vi "FuzzyEx Car Backward Parking.vi"() -> ()   [LabVIEW 2018]
doc: "本范例演示使用模糊逻辑在指定位置停车。"
uses:
  <vilib>/addons/Fuzzy Logic/TypeDefs/FL System.ctl
  <vilib>/addons/Fuzzy Logic/TypeDefs/FL Variable.ctl
  <vilib>/addons/Fuzzy Logic/TypeDefs/FL Membership Function.ctl
  <vilib>/addons/Fuzzy Logic/TypeDefs/FL Membership Function Shape.ctl
  <vilib>/addons/Fuzzy Logic/TypeDefs/FL Rule.ctl
  <vilib>/addons/Fuzzy Logic/TypeDefs/FL Antecedent.ctl
  <vilib>/addons/Fuzzy Logic/TypeDefs/FL Modifier.ctl
  <vilib>/addons/Fuzzy Logic/TypeDefs/FL Antecedent Connective.ctl
  <vilib>/addons/Fuzzy Logic/TypeDefs/FL Consequent.ctl
  <vilib>/addons/Fuzzy Logic/TypeDefs/FL Consequent Implication.ctl
  <vilib>/addons/Fuzzy Logic/TypeDefs/FL Defuzzification.ctl
  <vilib>/addons/Fuzzy Logic/TypeDefs/FL Interpolating polynomials.ctl
  <vilib>/addons/Fuzzy Logic/FL Fuzzy Controller (MISO).vi
  <vilib>/addons/Fuzzy Logic/NI_Fuzzy_Logic_API.lvlib
panel:
  out "反向模糊系统":T1={"input variables"=[{"name"="汽车-位置", "range"=[0.0, 10.0, 0.0, 10.0], "MFs"=[{"name"="左", "shape"=1, "points"=[0.0, 0.0, 1.0, 4.0], "color"=16711680, "user-defined shape index"=0}, {"name"="左-中", "shape"=0, "points"=[3.0, 4.0, 5.0], "color"=3342438, "user-defined shape index"=0}, {"name"="中", "shape"=0, "points"=[4.5, 5.0, 5.5], "color"=255, "user-defined shape index"=0}, {"name"="右-中", "shape"=0, "points"=[5.0, 6.0, 7.0], "color"=16724991, "user-defined shape index"=0}, {"name"="右", "shape"=1, "points"=[6.0, 9.0, 10.0, 10.0], "color"=26214, "user-defined shape index"=0}]}, {"name"="汽车-方向", "range"=[-90.0, 270.0, -90.0, 270.0], "MFs"=[{"name"="左-下", "shape"=1, "points"=[-90.0, -90.0, -45.0, 20.000000000000014], "color"=16711680, "user-defined shape index"=0}, {"name"="左", "shape"=0, "points"=[-20.000000000000014, 20.000000000000014, 70.0], "color"=3342438, "user-defined shape index"=0}, {"name"="左-上", "shape"=0, "points"=[45.0, 70.0, 90.0], "color"=16724991, "user-defined shape index"=0}, {"name"="上", "shape"=0, "points"=[75.0, 90.0, 104.99999999999999], "color"=255, "user-defined shape index"=0}, {"name"="右-上", "shape"=0, "points"=[90.0, 110.0, 135.0], "color"=10040064, "user-defined shape index"=0}, {"name"="右", "shape"=0, "points"=[110.0, 160.0, 200.0], "color"=13056, "user-defined shape index"=0}, {"name"="右-下", "shape"=1, "points"=[160.0, 225.0, 270.0, 270.0], "color"=26214, "user-defined shape index"=0}]}], "output variables"=[{"name"="转向-角", "range"=[-30.0, 30.0, -30.0, 30.0], "MFs"=[{"name"="负大", "shape"=0, "points"=[-30.0, -30.0, -15.0], "color"=16711680, "user-defined shape index"=0}, {"name"="负中间", "shape"=0, "points"=[-30.0, -15.0, -4.999999999999999], "color"=3342438, "user-defined shape index"=0}, {"name"="负小", "shape"=0, "points"=[-15.0, -4.999999999999999, 0.0], "color"=16724991, "user-defined shape index"=0}, {"name"="零", "shape"=0, "points"=[-4.999999999999999, 0.0, 5.000000000000002], "color"=255, "user-defined shape index"=0}, {"name"="正小", "shape"=0, "points"=[0.0, 5.000000000000002, 15.0], "color"=10040064, "user-defined shape index"=0}, {"name"="正中间", "shape"=0, "points"=[5.000000000000002, 15.0, 30.0], "color"=13056, "user-defined shape index"=0}, {"name"="正大", "shape"=0, "points"=[15.0, 30.0, 30.0], "color"=26214, "user-defined shape index"=0}]}], "rules"=[{"antecedents"=[{"Var Index"=0, "MF Index"=0, "Cond"=0}, {"Var Index"=1, "MF Index"=0, "Cond"=0}], "antecedent connective"=0, "consequents"=[{"Var Index"=0, "MF Index"=2, "Cond"=0}], "consequent implication"=0, "degree of support"=1.0}, {"antecedents"=[{"Var Index"=0, "MF Index"=0, "Cond"=0}, {"Var Index"=1, "MF Index"=1, "Cond"=0}], "antecedent connective"=0, "consequents"=[{"Var Index"=0, "MF Index"=4, "Cond"=0}], "consequent implication"=0, "degree of support"=1.0}, {"antecedents"=[{"Var Index"=0, "MF Index"=0, "Cond"=0}, {"Var Index"=1, "MF Index"=2, "Cond"=0}], "antecedent connective"=0, "consequents"=[{"Var Index"=0, "MF Index"=5, "Cond"=0}], "consequent implication"=0, "degree of support"=1.0}, {"antecedents"=[{"Var Index"=0, "MF Index"=0, "Cond"=0}, {"Var Index"=1, "MF Index"=3, "Cond"=0}], "antecedent connective"=0, "consequents"=[{"Var Index"=0, "MF Index"=5, "Cond"=0}], "consequent implication"=0, "degree of support"=1.0}, {"antecedents"=[{"Var Index"=0, "MF Index"=0, "Cond"=0}, {"Var Index"=1, "MF Index"=4, "Cond"=0}], "antecedent connective"=0, "consequents"=[{"Var Index"=0, "MF Index"=6, "Cond"=0}], "consequent implication"=0, "degree of support"=1.0}, {"antecedents"=[{"Var Index"=0, "MF Index"=0, "Cond"=0}, {"Var Index"=1, "MF Index"=5, "Cond"=0}], "antecedent connective"=0, "consequents"=[{"Var Index"=0, "MF Index"=6, "Cond"=0}], "consequent implication"=0, "degree of support"=1.0}, {"antecedents"=[{"Var Index"=0, "MF Index"=0, "Cond"=0}, {"Var Index"=1, "MF Index"=6, "Cond"=0}], "antecedent connective"=0, "consequents"=[{"Var Index"=0, "MF Index"=6, "Cond"=0}], "consequent implication"=0, "degree of support"=1.0}, {"antecedents"=[{"Var Index"=0, "MF Index"=1, "Cond"=0}, {"Var Index"=1, "MF Index"=0, "Cond"=0}], "antecedent connective"=0, "consequents"=[{"Var Index"=0, "MF Index"=1, "Cond"=0}], "consequent implication"=0, "degree of support"=1.0}, {"antecedents"=[{"Var Index"=0, "MF Index"=1, "Cond"=0}, {"Var Index"=1, "MF Index"=1, "Cond"=0}], "antecedent connective"=0, "consequents"=[{"Var Index"=0, "MF Index"=2, "Cond"=0}], "consequent implication"=0, "degree of support"=1.0}, {"antecedents"=[{"Var Index"=0, "MF Index"=1, "Cond"=0}, {"Var Index"=1, "MF Index"=2, "Cond"=0}], "antecedent connective"=0, "consequents"=[{"Var Index"=0, "MF Index"=4, "Cond"=0}], "consequent implication"=0, "degree of support"=1.0}, {"antecedents"=[{"Var Index"=0, "MF Index"=1, "Cond"=0}, {"Var Index"=1, "MF Index"=3, "Cond"=0}], "antecedent connective"=0, "consequents"=[{"Var Index"=0, "MF Index"=5, "Cond"=0}], "consequent implication"=0, "degree of support"=1.0}, {"antecedents"=[{"Var Index"=0, "MF Index"=1, "Cond"=0}, {"Var Index"=1, "MF Index"=4, "Cond"=0}], "antecedent connective"=0, "consequents"=[{"Var Index"=0, "MF Index"=5, "Cond"=0}], "consequent implication"=0, "degree of support"=1.0}, {"antecedents"=[{"Var Index"=0, "MF Index"=1, "Cond"=0}, {"Var Index"=1, "MF Index"=5, "Cond"=0}], "antecedent connective"=0, "consequents"=[{"Var Index"=0, "MF Index"=6, "Cond"=0}], "consequent implication"=0, "degree of support"=1.0}, {"antecedents"=[{"Var Index"=0, "MF Index"=1, "Cond"=0}, {"Var Index"=1, "MF Index"=6, "Cond"=0}], "antecedent connective"=0, "consequents"=[{"Var Index"=0, "MF Index"=6, "Cond"=0}], "consequent implication"=0, "degree of support"=1.0}, {"antecedents"=[{"Var Index"=0, "MF Index"=2, "Cond"=0}, {"Var Index"=1, "MF Index"=0, "Cond"=0}], "antecedent connective"=0, "consequents"=[{"Var Index"=0, "MF Index"=1, "Cond"=0}], "consequent implication"=0, "degree of support"=1.0}, {"antecedents"=[{"Var Index"=0, "MF Index"=2, "Cond"=0}, {"Var Index"=1, "MF Index"=1, "Cond"=0}], "antecedent connective"=0, "consequents"=[{"Var Index"=0, "MF Index"=1, "Cond"=0}], "consequent implication"=0, "degree of support"=1.0}, {"antecedents"=[{"Var Index"=0, "MF Index"=2, "Cond"=0}, {"Var Index"=1, "MF Index"=2, "Cond"=0}], "antecedent connective"=0, "consequents"=[{"Var Index"=0, "MF Index"=2, "Cond"=0}], "consequent implication"=0, "degree of support"=1.0}, {"antecedents"=[{"Var Index"=0, "MF Index"=2, "Cond"=0}, {"Var Index"=1, "MF Index"=3, "Cond"=0}], "antecedent connective"=0, "consequents"=[{"Var Index"=0, "MF Index"=3, "Cond"=0}], "consequent implication"=0, "degree of support"=1.0}, {"antecedents"=[{"Var Index"=0, "MF Index"=2, "Cond"=0}, {"Var Index"=1, "MF Index"=4, "Cond"=0}], "antecedent connective"=0, "consequents"=[{"Var Index"=0, "MF Index"=4, "Cond"=0}], "consequent implication"=0, "degree of support"=1.0}, {"antecedents"=[{"Var Index"=0, "MF Index"=2, "Cond"=0}, {"Var Index"=1, "MF Index"=5, "Cond"=0}], "antecedent connective"=0, "consequents"=[{"Var Index"=0, "MF Index"=5, "Cond"=0}], "consequent implication"=0, "degree of support"=1.0}, {"antecedents"=[{"Var Index"=0, "MF Index"=2, "Cond"=0}, {"Var Index"=1, "MF Index"=6, "Cond"=0}], "antecedent connective"=0, "consequents"=[{"Var Index"=0, "MF Index"=5, "Cond"=0}], "consequent implication"=0, "degree of support"=1.0}, {"antecedents"=[{"Var Index"=0, "MF Index"=3, "Cond"=0}, {"Var Index"=1, "MF Index"=0, "Cond"=0}], "antecedent connective"=0, "consequents"=[{"Var Index"=0, "MF Index"=0, "Cond"=0}], "consequent implication"=0, "degree of support"=1.0}, {"antecedents"=[{"Var Index"=0, "MF Index"=3, "Cond"=0}, {"Var Index"=1, "MF Index"=1, "Cond"=0}], "antecedent connective"=0, "consequents"=[{"Var Index"=0, "MF Index"=0, "Cond"=0}], "consequent implication"=0, "degree of support"=1.0}, {"antecedents"=[{"Var Index"=0, "MF Index"=3, "Cond"=0}, {"Var Index"=1, "MF Index"=2, "Cond"=0}], "antecedent connective"=0, "consequents"=[{"Var Index"=0, "MF Index"=0, "Cond"=0}], "consequent implication"=0, "degree of support"=1.0}, {"antecedents"=[{"Var Index"=0, "MF Index"=3, "Cond"=0}, {"Var Index"=1, "MF Index"=3, "Cond"=0}], "antecedent connective"=0, "consequents"=[{"Var Index"=0, "MF Index"=1, "Cond"=0}], "consequent implication"=0, "degree of support"=1.0}, {"antecedents"=[{"Var Index"=0, "MF Index"=3, "Cond"=0}, {"Var Index"=1, "MF Index"=4, "Cond"=0}], "antecedent connective"=0, "consequents"=[{"Var Index"=0, "MF Index"=1, "Cond"=0}], "consequent implication"=0, "degree of support"=1.0}, {"antecedents"=[{"Var Index"=0, "MF Index"=3, "Cond"=0}, {"Var Index"=1, "MF Index"=5, "Cond"=0}], "antecedent connective"=0, "consequents"=[{"Var Index"=0, "MF Index"=2, "Cond"=0}], "consequent implication"=0, "degree of support"=1.0}, {"antecedents"=[{"Var Index"=0, "MF Index"=3, "Cond"=0}, {"Var Index"=1, "MF Index"=6, "Cond"=0}], "antecedent connective"=0, "consequents"=[{"Var Index"=0, "MF Index"=2, "Cond"=0}], "consequent implication"=0, "degree of support"=1.0}, {"antecedents"=[{"Var Index"=0, "MF Index"=4, "Cond"=0}, {"Var Index"=1, "MF Index"=0, "Cond"=0}], "antecedent connective"=0, "consequents"=[{"Var Index"=0, "MF Index"=0, "Cond"=0}], "consequent implication"=0, "degree of support"=1.0}, {"antecedents"=[{"Var Index"=0, "MF Index"=4, "Cond"=0}, {"Var Index"=1, "MF Index"=1, "Cond"=0}], "antecedent connective"=0, "consequents"=[{"Var Index"=0, "MF Index"=0, "Cond"=0}], "consequent implication"=0, "degree of support"=1.0}, {"antecedents"=[{"Var Index"=0, "MF Index"=4, "Cond"=0}, {"Var Index"=1, "MF Index"=2, "Cond"=0}], "antecedent connective"=0, "consequents"=[{"Var Index"=0, "MF Index"=0, "Cond"=0}], "consequent implication"=0, "degree of support"=1.0}, {"antecedents"=[{"Var Index"=0, "MF Index"=4, "Cond"=0}, {"Var Index"=1, "MF Index"=3, "Cond"=0}], "antecedent connective"=0, "consequents"=[{"Var Index"=0, "MF Index"=1, "Cond"=0}], "consequent implication"=0, "degree of support"=1.0}, {"antecedents"=[{"Var Index"=0, "MF Index"=4, "Cond"=0}, {"Var Index"=1, "MF Index"=4, "Cond"=0}], "antecedent connective"=0, "consequents"=[{"Var Index"=0, "MF Index"=1, "Cond"=0}], "consequent implication"=0, "degree of support"=1.0}, {"antecedents"=[{"Var Index"=0, "MF Index"=4, "Cond"=0}, {"Var Index"=1, "MF Index"=5, "Cond"=0}], "antecedent connective"=0, "consequents"=[{"Var Index"=0, "MF Index"=2, "Cond"=0}], "consequent implication"=0, "degree of support"=1.0}, {"antecedents"=[{"Var Index"=0, "MF Index"=4, "Cond"=0}, {"Var Index"=1, "MF Index"=6, "Cond"=0}], "antecedent connective"=0, "consequents"=[{"Var Index"=0, "MF Index"=2, "Cond"=0}], "consequent implication"=0, "degree of support"=1.0}], "defuzzification method"=0, "description"="用于自动操控过程的双输入模糊控制器从反方向的任意起始位置到装载坡道引导卡车。卡车运行在恒定低速。\n\n操控算法由适当的规则库（基础知识）表示。\n\n当前操控情况至少由两个语言输入变量：相对装载坡道位置的“车辆-位置”和“车辆-方向”表示。\n\n控制器的输出变量“转向-角”作为过程控制变量。\n\n该模糊控制器负责普通反向操控操作。", "user MF interpolating polynomials"=[]} {"user MF interpolating polynomials"."coa_x(y) coeff" format="%.4g"; "user MF interpolating polynomials"."Area(y) coeff" format="%.4g"; "user MF interpolating polynomials"."X(y) coeff" format="%.4g"; "user MF interpolating polynomials"."Y(x) coeff" format="%.4g"; "user MF interpolating polynomials"."Y" format="%.4g"; "user MF interpolating polynomials"."X" format="%.4g"; "defuzzification method" items=["面积中心", "改进面积中心", "和中心", "最大值中心", "最大值平均"]; "rules"."consequents"."Var Index" min=0; "rules"."consequents"."Cond" items=["=", "!="]; "rules"."consequents"."MF Index" min=0; "rules"."antecedents"."Var Index" min=0; "rules"."antecedents"."Cond" items=["=", "!="]; "rules"."antecedents"."MF Index" min=0; "rules"."consequent implication" items=["最小值", "乘积"]; "rules"."antecedent connective" items=["与（最小值）", "与（乘积）", "或（最大值）", "或（概率方法）"]; "output variables"."MFs"."shape" items=["三角形", "梯形", "单元素", "S形", "高斯形", "用户定义"]; "input variables"."MFs"."shape" items=["三角形", "梯形", "单元素", "S形", "高斯形", "用户定义"]}
  out "正向模糊系统":T1={"input variables"=[{"name"="汽车-位置", "range"=[0.0, 10.0, 0.0, 10.0], "MFs"=[{"name"="左", "shape"=1, "points"=[0.0, 0.0, 1.0, 4.0], "color"=16711680, "user-defined shape index"=0}, {"name"="左-中", "shape"=0, "points"=[3.0, 4.0, 5.0], "color"=3342438, "user-defined shape index"=0}, {"name"="中", "shape"=0, "points"=[4.5, 5.0, 5.5], "color"=255, "user-defined shape index"=0}, {"name"="右-中", "shape"=0, "points"=[5.0, 6.0, 7.0], "color"=16724991, "user-defined shape index"=0}, {"name"="右", "shape"=1, "points"=[6.0, 9.0, 10.0, 10.0], "color"=26214, "user-defined shape index"=0}]}, {"name"="汽车-方向", "range"=[-90.0, 270.0, -90.0, 270.0], "MFs"=[{"name"="左-下", "shape"=1, "points"=[-90.0, -90.0, -45.0, 20.000000000000014], "color"=16711680, "user-defined shape index"=0}, {"name"="左", "shape"=0, "points"=[-20.000000000000014, 20.000000000000014, 70.0], "color"=3342438, "user-defined shape index"=0}, {"name"="左-上", "shape"=0, "points"=[45.0, 70.0, 90.0], "color"=16724991, "user-defined shape index"=0}, {"name"="上", "shape"=0, "points"=[75.0, 90.0, 104.99999999999999], "color"=255, "user-defined shape index"=0}, {"name"="右-上", "shape"=0, "points"=[90.0, 110.0, 135.0], "color"=10040064, "user-defined shape index"=0}, {"name"="右", "shape"=0, "points"=[110.0, 160.0, 200.0], "color"=13056, "user-defined shape index"=0}, {"name"="右-下", "shape"=1, "points"=[160.0, 225.0, 270.0, 270.0], "color"=26214, "user-defined shape index"=0}]}], "output variables"=[{"name"="转向-角", "range"=[-30.0, 30.0, -30.0, 30.0], "MFs"=[{"name"="负大", "shape"=0, "points"=[-30.0, -30.0, -15.0], "color"=16711680, "user-defined shape index"=0}, {"name"="负中间", "shape"=0, "points"=[-30.0, -15.0, -4.999999999999999], "color"=3342438, "user-defined shape index"=0}, {"name"="负小", "shape"=0, "points"=[-15.0, -4.999999999999999, 0.0], "color"=16724991, "user-defined shape index"=0}, {"name"="零", "shape"=0, "points"=[-4.999999999999999, 0.0, 5.000000000000002], "color"=255, "user-defined shape index"=0}, {"name"="正小", "shape"=0, "points"=[0.0, 5.000000000000002, 15.0], "color"=10040064, "user-defined shape index"=0}, {"name"="正中间", "shape"=0, "points"=[5.000000000000002, 15.0, 30.0], "color"=13056, "user-defined shape index"=0}, {"name"="正大", "shape"=0, "points"=[15.0, 30.0, 30.0], "color"=26214, "user-defined shape index"=0}]}], "rules"=[{"antecedents"=[{"Var Index"=0, "MF Index"=0, "Cond"=0}, {"Var Index"=1, "MF Index"=0, "Cond"=0}], "antecedent connective"=0, "consequents"=[{"Var Index"=0, "MF Index"=6, "Cond"=0}], "consequent implication"=0, "degree of support"=1.0}, {"antecedents"=[{"Var Index"=0, "MF Index"=0, "Cond"=0}, {"Var Index"=1, "MF Index"=1, "Cond"=0}], "antecedent connective"=0, "consequents"=[{"Var Index"=0, "MF Index"=6, "Cond"=0}], "consequent implication"=0, "degree of support"=1.0}, {"antecedents"=[{"Var Index"=0, "MF Index"=0, "Cond"=0}, {"Var Index"=1, "MF Index"=2, "Cond"=0}], "antecedent connective"=0, "consequents"=[{"Var Index"=0, "MF Index"=5, "Cond"=0}], "consequent implication"=0, "degree of support"=1.0}, {"antecedents"=[{"Var Index"=0, "MF Index"=0, "Cond"=0}, {"Var Index"=1, "MF Index"=3, "Cond"=0}], "antecedent connective"=0, "consequents"=[{"Var Index"=0, "MF Index"=5, "Cond"=0}], "consequent implication"=0, "degree of support"=1.0}, {"antecedents"=[{"Var Index"=0, "MF Index"=0, "Cond"=0}, {"Var Index"=1, "MF Index"=4, "Cond"=0}], "antecedent connective"=0, "consequents"=[{"Var Index"=0, "MF Index"=4, "Cond"=0}], "consequent implication"=0, "degree of support"=1.0}, {"antecedents"=[{"Var Index"=0, "MF Index"=0, "Cond"=0}, {"Var Index"=1, "MF Index"=5, "Cond"=0}], "antecedent connective"=0, "consequents"=[{"Var Index"=0, "MF Index"=2, "Cond"=0}], "consequent implication"=0, "degree of support"=1.0}, {"antecedents"=[{"Var Index"=0, "MF Index"=0, "Cond"=0}, {"Var Index"=1, "MF Index"=6, "Cond"=0}], "antecedent connective"=0, "consequents"=[{"Var Index"=0, "MF Index"=0, "Cond"=0}], "consequent implication"=0, "degree of support"=1.0}, {"antecedents"=[{"Var Index"=0, "MF Index"=1, "Cond"=0}, {"Var Index"=1, "MF Index"=0, "Cond"=0}], "antecedent connective"=0, "consequents"=[{"Var Index"=0, "MF Index"=6, "Cond"=0}], "consequent implication"=0, "degree of support"=1.0}, {"antecedents"=[{"Var Index"=0, "MF Index"=1, "Cond"=0}, {"Var Index"=1, "MF Index"=1, "Cond"=0}], "antecedent connective"=0, "consequents"=[{"Var Index"=0, "MF Index"=6, "Cond"=0}], "consequent implication"=0, "degree of support"=1.0}, {"antecedents"=[{"Var Index"=0, "MF Index"=1, "Cond"=0}, {"Var Index"=1, "MF Index"=2, "Cond"=0}], "antecedent connective"=0, "consequents"=[{"Var Index"=0, "MF Index"=5, "Cond"=0}], "consequent implication"=0, "degree of support"=1.0}, {"antecedents"=[{"Var Index"=0, "MF Index"=1, "Cond"=0}, {"Var Index"=1, "MF Index"=3, "Cond"=0}], "antecedent connective"=0, "consequents"=[{"Var Index"=0, "MF Index"=5, "Cond"=0}], "consequent implication"=0, "degree of support"=1.0}, {"antecedents"=[{"Var Index"=0, "MF Index"=1, "Cond"=0}, {"Var Index"=1, "MF Index"=4, "Cond"=0}], "antecedent connective"=0, "consequents"=[{"Var Index"=0, "MF Index"=4, "Cond"=0}], "consequent implication"=0, "degree of support"=1.0}, {"antecedents"=[{"Var Index"=0, "MF Index"=1, "Cond"=0}, {"Var Index"=1, "MF Index"=5, "Cond"=0}], "antecedent connective"=0, "consequents"=[{"Var Index"=0, "MF Index"=2, "Cond"=0}], "consequent implication"=0, "degree of support"=1.0}, {"antecedents"=[{"Var Index"=0, "MF Index"=1, "Cond"=0}, {"Var Index"=1, "MF Index"=6, "Cond"=0}], "antecedent connective"=0, "consequents"=[{"Var Index"=0, "MF Index"=1, "Cond"=0}], "consequent implication"=0, "degree of support"=1.0}, {"antecedents"=[{"Var Index"=0, "MF Index"=2, "Cond"=0}, {"Var Index"=1, "MF Index"=0, "Cond"=0}], "antecedent connective"=0, "consequents"=[{"Var Index"=0, "MF Index"=5, "Cond"=0}], "consequent implication"=0, "degree of support"=1.0}, {"antecedents"=[{"Var Index"=0, "MF Index"=2, "Cond"=0}, {"Var Index"=1, "MF Index"=1, "Cond"=0}], "antecedent connective"=0, "consequents"=[{"Var Index"=0, "MF Index"=5, "Cond"=0}], "consequent implication"=0, "degree of support"=1.0}, {"antecedents"=[{"Var Index"=0, "MF Index"=2, "Cond"=0}, {"Var Index"=1, "MF Index"=2, "Cond"=0}], "antecedent connective"=0, "consequents"=[{"Var Index"=0, "MF Index"=4, "Cond"=0}], "consequent implication"=0, "degree of support"=1.0}, {"antecedents"=[{"Var Index"=0, "MF Index"=2, "Cond"=0}, {"Var Index"=1, "MF Index"=3, "Cond"=0}], "antecedent connective"=0, "consequents"=[{"Var Index"=0, "MF Index"=3, "Cond"=0}], "consequent implication"=0, "degree of support"=1.0}, {"antecedents"=[{"Var Index"=0, "MF Index"=2, "Cond"=0}, {"Var Index"=1, "MF Index"=4, "Cond"=0}], "antecedent connective"=0, "consequents"=[{"Var Index"=0, "MF Index"=2, "Cond"=0}], "consequent implication"=0, "degree of support"=1.0}, {"antecedents"=[{"Var Index"=0, "MF Index"=2, "Cond"=0}, {"Var Index"=1, "MF Index"=5, "Cond"=0}], "antecedent connective"=0, "consequents"=[{"Var Index"=0, "MF Index"=1, "Cond"=0}], "consequent implication"=0, "degree of support"=1.0}, {"antecedents"=[{"Var Index"=0, "MF Index"=2, "Cond"=0}, {"Var Index"=1, "MF Index"=6, "Cond"=0}], "antecedent connective"=0, "consequents"=[{"Var Index"=0, "MF Index"=1, "Cond"=0}], "consequent implication"=0, "degree of support"=1.0}, {"antecedents"=[{"Var Index"=0, "MF Index"=3, "Cond"=0}, {"Var Index"=1, "MF Index"=0, "Cond"=0}], "antecedent connective"=0, "consequents"=[{"Var Index"=0, "MF Index"=5, "Cond"=0}], "consequent implication"=0, "degree of support"=1.0}, {"antecedents"=[{"Var Index"=0, "MF Index"=3, "Cond"=0}, {"Var Index"=1, "MF Index"=1, "Cond"=0}], "antecedent connective"=0, "consequents"=[{"Var Index"=0, "MF Index"=4, "Cond"=0}], "consequent implication"=0, "degree of support"=1.0}, {"antecedents"=[{"Var Index"=0, "MF Index"=3, "Cond"=0}, {"Var Index"=1, "MF Index"=2, "Cond"=0}], "antecedent connective"=0, "consequents"=[{"Var Index"=0, "MF Index"=2, "Cond"=0}], "consequent implication"=0, "degree of support"=1.0}, {"antecedents"=[{"Var Index"=0, "MF Index"=3, "Cond"=0}, {"Var Index"=1, "MF Index"=3, "Cond"=0}], "antecedent connective"=0, "consequents"=[{"Var Index"=0, "MF Index"=1, "Cond"=0}], "consequent implication"=0, "degree of support"=1.0}, {"antecedents"=[{"Var Index"=0, "MF Index"=3, "Cond"=0}, {"Var Index"=1, "MF Index"=4, "Cond"=0}], "antecedent connective"=0, "consequents"=[{"Var Index"=0, "MF Index"=1, "Cond"=0}], "consequent implication"=0, "degree of support"=1.0}, {"antecedents"=[{"Var Index"=0, "MF Index"=3, "Cond"=0}, {"Var Index"=1, "MF Index"=5, "Cond"=0}], "antecedent connective"=0, "consequents"=[{"Var Index"=0, "MF Index"=0, "Cond"=0}], "consequent implication"=0, "degree of support"=1.0}, {"antecedents"=[{"Var Index"=0, "MF Index"=3, "Cond"=0}, {"Var Index"=1, "MF Index"=6, "Cond"=0}], "antecedent connective"=0, "consequents"=[{"Var Index"=0, "MF Index"=0, "Cond"=0}], "consequent implication"=0, "degree of support"=1.0}, {"antecedents"=[{"Var Index"=0, "MF Index"=4, "Cond"=0}, {"Var Index"=1, "MF Index"=0, "Cond"=0}], "antecedent connective"=0, "consequents"=[{"Var Index"=0, "MF Index"=5, "Cond"=0}], "consequent implication"=0, "degree of support"=1.0}, {"antecedents"=[{"Var Index"=0, "MF Index"=4, "Cond"=0}, {"Var Index"=1, "MF Index"=1, "Cond"=0}], "antecedent connective"=0, "consequents"=[{"Var Index"=0, "MF Index"=4, "Cond"=0}], "consequent implication"=0, "degree of support"=1.0}, {"antecedents"=[{"Var Index"=0, "MF Index"=4, "Cond"=0}, {"Var Index"=1, "MF Index"=2, "Cond"=0}], "antecedent connective"=0, "consequents"=[{"Var Index"=0, "MF Index"=2, "Cond"=0}], "consequent implication"=0, "degree of support"=1.0}, {"antecedents"=[{"Var Index"=0, "MF Index"=4, "Cond"=0}, {"Var Index"=1, "MF Index"=3, "Cond"=0}], "antecedent connective"=0, "consequents"=[{"Var Index"=0, "MF Index"=1, "Cond"=0}], "consequent implication"=0, "degree of support"=1.0}, {"antecedents"=[{"Var Index"=0, "MF Index"=4, "Cond"=0}, {"Var Index"=1, "MF Index"=4, "Cond"=0}], "antecedent connective"=0, "consequents"=[{"Var Index"=0, "MF Index"=1, "Cond"=0}], "consequent implication"=0, "degree of support"=1.0}, {"antecedents"=[{"Var Index"=0, "MF Index"=4, "Cond"=0}, {"Var Index"=1, "MF Index"=5, "Cond"=0}], "antecedent connective"=0, "consequents"=[{"Var Index"=0, "MF Index"=0, "Cond"=0}], "consequent implication"=0, "degree of support"=1.0}, {"antecedents"=[{"Var Index"=0, "MF Index"=4, "Cond"=0}, {"Var Index"=1, "MF Index"=6, "Cond"=0}], "antecedent connective"=0, "consequents"=[{"Var Index"=0, "MF Index"=0, "Cond"=0}], "consequent implication"=0, "degree of support"=1.0}], "defuzzification method"=0, "description"="用于自动操控过程的双输入模糊控制器从反方向的任意起始位置到装载坡道引导卡车。卡车运行在恒定低速。\n\n操控算法由适当的规则库（基础知识）表示。\n\n当前操控情况至少由两个语言输入变量：相对装载坡道位置的“车辆-位置”和“车辆-方向”表示。\n\n控制器的输出变量“转向-角”作为过程控制变量。\n\n当反向操作不能使车辆上坡道时，该模糊控制器负责前向操控操作，让车辆处在正确的开始位置。 ", "user MF interpolating polynomials"=[]} {"user MF interpolating polynomials"."coa_x(y) coeff" format="%.4g"; "user MF interpolating polynomials"."Area(y) coeff" format="%.4g"; "user MF interpolating polynomials"."X(y) coeff" format="%.4g"; "user MF interpolating polynomials"."Y(x) coeff" format="%.4g"; "user MF interpolating polynomials"."Y" format="%.4g"; "user MF interpolating polynomials"."X" format="%.4g"; "defuzzification method" items=["面积中心", "改进面积中心", "和中心", "最大值中心", "最大值平均"]; "rules"."consequents"."Var Index" min=0; "rules"."consequents"."Cond" items=["=", "!="]; "rules"."consequents"."MF Index" min=0; "rules"."antecedents"."Var Index" min=0; "rules"."antecedents"."Cond" items=["=", "!="]; "rules"."antecedents"."MF Index" min=0; "rules"."consequent implication" items=["最小值", "乘积"]; "rules"."antecedent connective" items=["与（最小值）", "与（乘积）", "或（最大值）", "或（概率方法）"]; "output variables"."MFs"."shape" items=["三角形", "梯形", "单元素", "S形", "高斯形", "用户定义"]; "input variables"."MFs"."shape" items=["三角形", "梯形", "单元素", "S形", "高斯形", "用户定义"]}
  in  "激活模糊控制器":bool
  out "转向角":picture
  out "到达":bool
  out "方向盘":dbl
  in  "初始车辆角度":dbl(knob)=-56.0 min=-90.0 max=270.0 step=1.0 scale=-90.0..270.0
  in  "停止":bool
  out "网格":cluster{dbl[], dbl[]}[](graph)
  out "停车":picture
  # "概述：本范例演示使用模糊逻辑模拟在指定位置停车。\n操作步骤：\n1.运行VI。\n2.移动游标，设置车辆初始位置和初始车辆角度。\n3.单击激活模糊控制器，使用模糊逻辑停车，并确认车辆倒至车库。\n4.单击停止按钮停止VI。"
  # "车库"
  # "IF"
  # "THEN"
  # "IF"
  # "THEN"
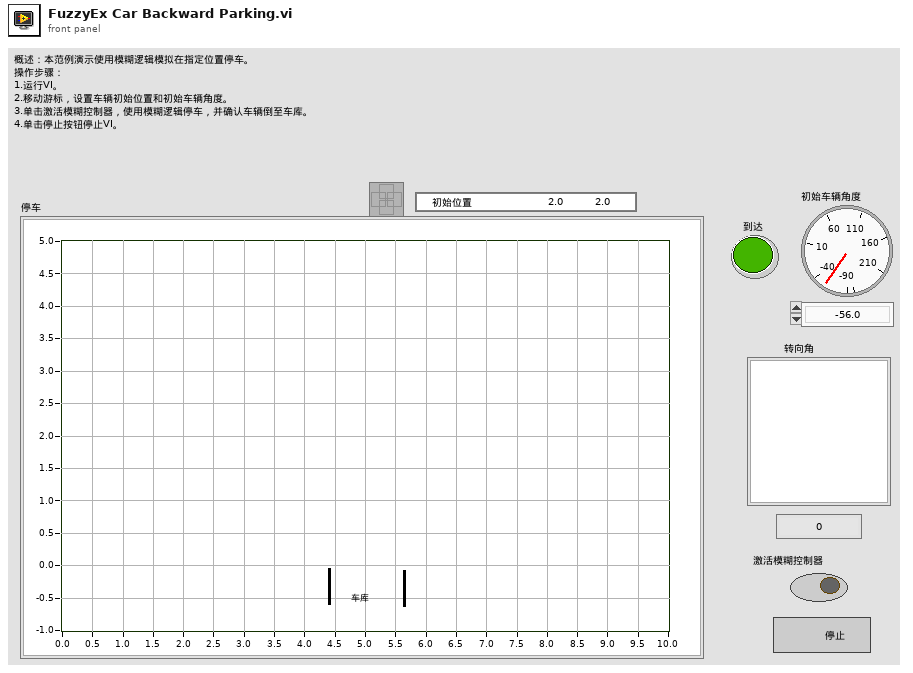
[diagram p1: front panel]
types:
  T1 = typedef "NI_Fuzzy_Logic_API.lvlib/FL System.ctl" = cluster{"input variables":T2[], "output variables":T2[], "rules":T5[], "defuzzification method":T11, "description":string, "user MF interpolating polynomials":T12[]}
  T2 = typedef "NI_Fuzzy_Logic_API.lvlib/FL Variable.ctl" = cluster{"name":string, "range":dbl[], "MFs":T3[]}
  T3 = typedef "NI_Fuzzy_Logic_API.lvlib/FL Membership Function.ctl" = cluster{"name":string, "shape":T4, "points":dbl[], "color":u32, "user-defined shape index":i32}
  T4 = typedef "NI_Fuzzy_Logic_API.lvlib/FL Membership Function Shape.ctl" = u16
  T5 = typedef "NI_Fuzzy_Logic_API.lvlib/FL Rule.ctl" = cluster{"antecedents":T6[], "antecedent connective":T8, "consequents":T9[], "consequent implication":T10, "degree of support":dbl}
  T6 = typedef "NI_Fuzzy_Logic_API.lvlib/FL Antecedent.ctl" = cluster{"Var Index":i32, "MF Index":i32, "Cond":T7}
  T7 = typedef "NI_Fuzzy_Logic_API.lvlib/FL Modifier.ctl" = u16
  T8 = typedef "NI_Fuzzy_Logic_API.lvlib/FL Antecedent Connective.ctl" = u16
  T9 = typedef "NI_Fuzzy_Logic_API.lvlib/FL Consequent.ctl" = cluster{"Var Index":i32, "MF Index":i32, "Cond":T7}
  T10 = typedef "NI_Fuzzy_Logic_API.lvlib/FL Consequent Implication.ctl" = u16
  T11 = typedef "NI_Fuzzy_Logic_API.lvlib/FL Defuzzification.ctl" = u16
  T12 = typedef "NI_Fuzzy_Logic_API.lvlib/FL Interpolating polynomials.ctl" = cluster{"X":dbl[], "Y":dbl[], "Y(x) coeff":dbl[][], "X(y) coeff":dbl[][], "Area(y) coeff":dbl[][], "coa_x(y) coeff":dbl[][]}
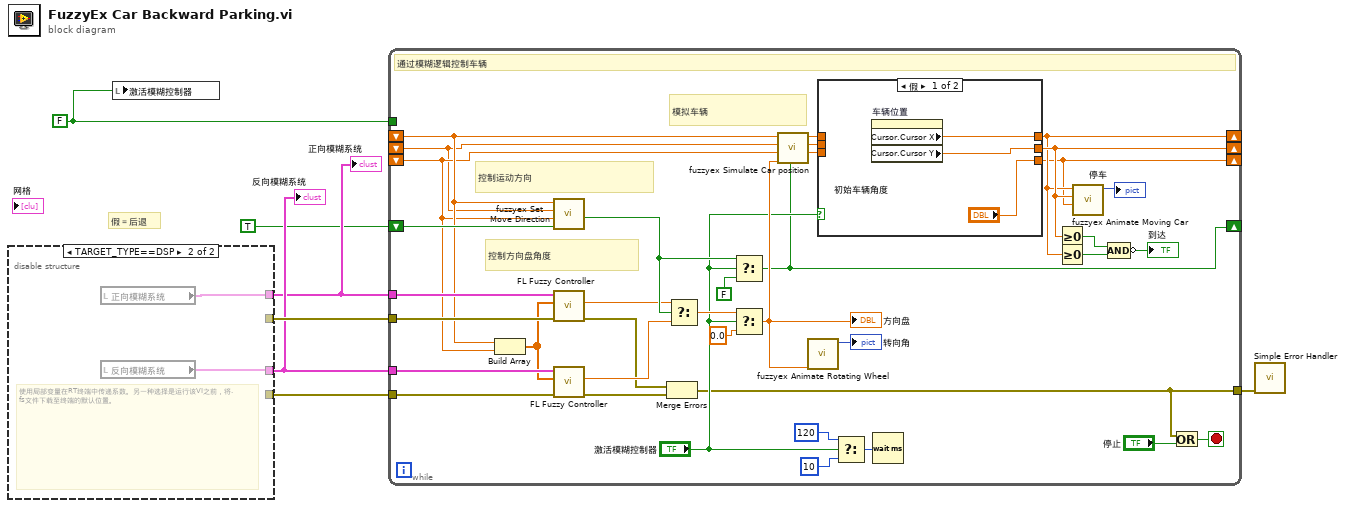
[diagram p0: block diagram]
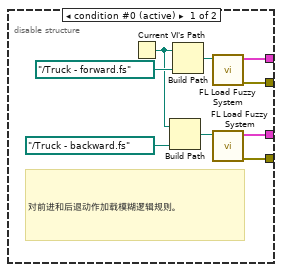
[diagram p2: hidden frame]
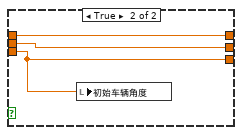
[diagram p3: hidden frame]
diagram:
  w3 = FALSE ("Operation Mode")
  # "假＝后退"
  n1 = disable-structure "Conditional Disable Structure" shown="TARGET_TYPE==DSP" {
    disable-tunnel: [w16 _] -> w7
    disable-tunnel: [w11 _] -> w6
    disable-tunnel: [w10 w17] -> w5
    disable-tunnel: [w9 w18] -> w4
    frame condition #0 (active) {
      # "对前进和后退动作加载模糊逻辑规则。"
      n2 = Current VI's Path() -> (path=w8:path)
      n3 = Build Path(base path=w8, name or relative path=path "../Truck - backward.fs") -> (appended path=w14:path)
      n4 = Build Path(base path=w8, name or relative path=path "../Truck - forward.fs") -> (appended path=w15:path)
      n5 = call <vilib>:"FL Load Fuzzy System.vi"("file path"=w15) -> ("error out"=w16:errorcluster, "fuzzy system out"=w9:T1)  [unwired: 1 in, 8 out]
      n6 = call <vilib>:"FL Load Fuzzy System.vi"("file path"=w14) -> ("error out"=w11:errorcluster, "fuzzy system out"=w10:T1)  [unwired: 1 in, 8 out]
    }
    frame condition #1 {
      # "使用局部变量在RT终端中传递系数。另一种选择是运行该VI之前，将.fs文件下载至终端的默认位置。"
      n7 = local read "正向模糊系统"() -> (w18:T1)
      n8 = local read "反向模糊系统"() -> (w17:T1)
    }
  }
  "正向模糊系统" <- w4
  "反向模糊系统" <- w5
  n9 = local write "激活模糊控制器"(w3) -> ()
  n10 = while {
    tunnel: w7 -> [w48]
    tunnel: w4 -> [w49]
    shift-left: TRUE -> [w52]
    shift-right: [w22] -> _
    shift-left: _ -> [w45]
    shift-right: [w42] -> _
    shift-left: _ -> [w24]
    shift-right: [w39] -> _
    shift-left: _ -> [w23]
    shift-right: [w43] -> _
    tunnel: w3 -> [_]
    tunnel: w5 -> [w44]
    tunnel: w6 -> [w35]
    tunnel: [w28] -> w2
    stop <- w27 stop-if-true
    # "控制方向盘角度"
    # "模拟车辆"
    # "控制运动方向"
    # "通过模糊逻辑控制车辆"
    n11 = Build Array(w45, w24) -> (w34:dbl[])
    n12 = call "fuzzyex Set Move Direction.vi"("direction"=w52, "beta"=w24, "y(VC)"=w23, "x(VC)"=w45) -> ("New Dir"=w40:bool)
    n13 = call-poly <vilib>:"FL Fuzzy Controller.vi"("error in (no error)"=w48, "input values"=w34, "fuzzy system in"=w49) -> ("error out"=w30:errorcluster, "output value"=w33:dbl)  [unwired: 7 out]
    n14 = call-poly <vilib>:"FL Fuzzy Controller.vi"("error in (no error)"=w35, "input values"=w34, "fuzzy system in"=w44) -> ("error out"=w29:errorcluster, "output value"=w32:dbl)  [unwired: 7 out]
    n15 = Merge Errors(w30, w29) -> (w28:errorcluster)
    n16 = Select(t=w33, s=w40, f=w32) -> (s? t:f=w51:dbl)
    n17 = Select(t=w40, s="激活模糊控制器", f=FALSE) -> (s? t:f=w22:bool)
    n18 = Select(t=w51, s="激活模糊控制器", f=0.0) -> (s? t:f=w47:dbl)
    "方向盘" <- w47
    n19 = call "fuzzyex Simulate Car position.vi"("Direction"=w22, "Steering Angle (Phi)"=w47, "Current Vehicle Orientation (Beta)"=w24, "Current Position Y"=w23, "Current Position X"=w45) -> ("New Vehicle Orientation Beta"=w36:dbl, "New position Y"=w37:dbl, "New position X"=w38:dbl)  [unwired: 2 out]
    n20 = call "fuzzyex Animate Rotating Wheel.vi"("Angle (deg)"=w47) -> ("new picture"=→"转向角":picture)  [unwired: 10 out]
    n21 = case shown="假" "激活模糊控制器" {
      tunnel: w37 -> [_ w60]
      tunnel: w38 -> [_ w61]
      tunnel: w36 -> [_ w59]
      tunnel: [w56 w60] -> w43
      tunnel: [w58 w61] -> w42
      tunnel: ["初始车辆角度" w59] -> w39
      frame False {
        n22 = property on="车辆位置" class="XYGraph (严格)"() -> ("Cursor.Cursor X"=w58:dbl, "Cursor.Cursor Y"=w56:dbl)  [unwired: 2 in, 2 out]
      }
      frame True {
        n23 = local write "初始车辆角度"(w59) -> ()
      }
    }
    n24 = Select(t=u32 120, s="激活模糊控制器", f=u32 10) -> (s? t:f=w55:u32)
    n25 = Wait (ms)(milliseconds to wait=w55) -> ()  [unwired: 1 out]
    n26 = Greater Or Equal To 0?(x=w43) -> (x >= 0?=w54:bool)
    n27 = Greater Or Equal To 0?(x=w42) -> (x >= 0?=w53:bool)
    n28 = call "fuzzyex Animate Moving Car.vi"("Car Angle (deg)"=w39, "y position"=w43, "x position"=w42) -> ("new picture"=→"停车":picture)  [unwired: 8 out]
    n29 = Compound Arithmetic op=AND(w54, w53) -> (invert →"到达":bool)
    n30 = Or(x=w28, y="停止") -> (x .or. y?=w27:bool)
  }
  n31 = call <vilib>:"Simple Error Handler.vi"("error in (no error)"=w2) -> ()  [unwired: 4 in, 5 out]
